vi "check_if_top_level_vi_is_running.vi"(8 "error in (no error)":errorcluster) -> (0 "error out":errorcluster, 3 "stop?":bool)   [LabVIEW 2014]
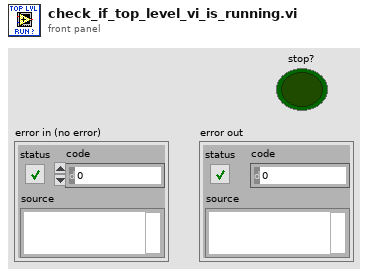
[diagram p1: front panel]
types:
  T1 = enum32{"Bad", "Idle", "Run top level", "Running"}
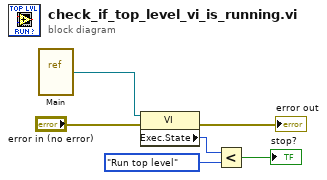
[diagram p0: block diagram]
diagram:
  n1 = vi-ref "Main.vi"() -> (w1:refnum<vi>)
  n2 = property class="VI"(reference=w1, error in="error in (no error)") -> (error out=→"error out":errorcluster, "Exec.State"=w2:T1)  [unwired: 1 out]
  n3 = Less?(x=w2, y=T1."Run top level") -> (x < y?=→"stop?":bool)
